vi "TWM Client Wait ACK.vi"(5 "timeout [ms] (3000)":i32=3000, 7 "key string":string="TWM:command:EndOfPacket", 8 "error in":errorcluster, 10 "command header":string, 11 "handle":i32) -> (0 "error out":errorcluster, 3 "handle out":i32)   [LabVIEW 2020, in "TWM Client.lvlib"]
doc: "Wait for ACK message from server."
uses:
  TWM Client.lvlib
  octave/infolib/infolib.lvlib
  <vilib>/ErrorRing/Error Ring.xnode
  <vilib>/Utility/error.llb/Error Cluster From Error Code.vi
  octave/infolib/Get 1D String.vi
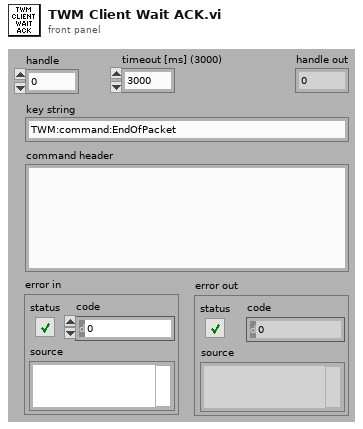
[diagram p1: front panel]
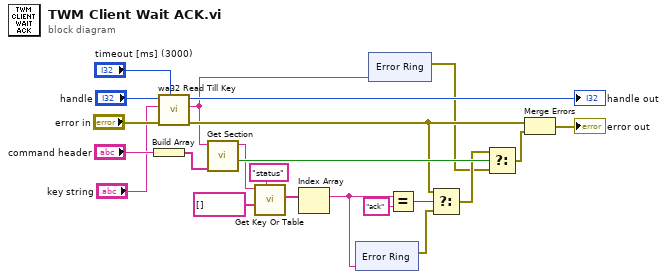
[diagram p0: block diagram]
diagram:
  n1 = Build Array("command header") -> (w1:string[])
  n2 = call "wa32 Read Till Key.vi"("timeout [ms] (1000)"="timeout [ms] (3000)", "error in"="error in", "key string"="key string", "handle"="handle") -> ("error out"=w11:errorcluster, "read message"=w5:string, "handle out"=→"handle out":i32)  [unwired: 5 in]
  n3 = call "Get Section.vi"("sections"=w1, "info data"=w5) -> ("exist"=w17:bool, "section part"=w16:string)  [unwired: 7 in, 1 out]
  n4 = call-poly "Get Key Or Table.vi"("key description"="status", "string"=string[] [], "info data"=w16) -> ("value"=w8:string[])  [unwired: 5 in, 3 out]
  n5 = Index Array(array=w8) -> (element=w3:string)  [unwired: 1 in]
  n6 = xnode "Error Ring"("parameter 0"=w3) -> ("error out"=w7:errorcluster)
  n7 = xnode "Error Ring"("parameter 0"=w5) -> ("error out"=w6:errorcluster)
  n8 = Equal?(x=w3, y="ack") -> (x = y?=w13:bool)
  n9 = Select(t=w11, s=w13, f=w7) -> (s? t:f=w12:errorcluster)
  n10 = Select(t=w12, s=w17, f=w6) -> (s? t:f=w10:errorcluster)
  n11 = Merge Errors(w11, w10) -> (→"error out":errorcluster)
